vi "Append Dictionary.vi"(8 "error in (no error)":errorcluster, 10 "key-value":T1, 11 "Control Experiment":refnum<class "Control Experiment.lvclass">) -> (0 "error out":errorcluster, 3 "Control Experiment out":refnum<class "Control Experiment.lvclass">)   [LabVIEW 2016, in "Control Experiment.lvclass"]
uses:
  Control Experiment.lvclass
  <userlib>/LevyLab/LV to ITX/Data/Typedefs/Dictionary--cluster.ctl
  <userlib>/LevyLab/LV to ITX/Data/Data.lvclass
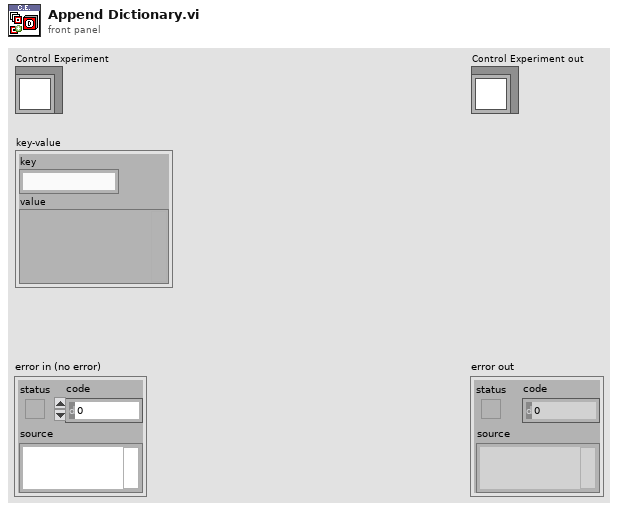
[diagram p1: front panel]
types:
  T1 = typedef "Data.lvclass/Dictionary--cluster.ctl" = cluster{"key":string, "value":variant}
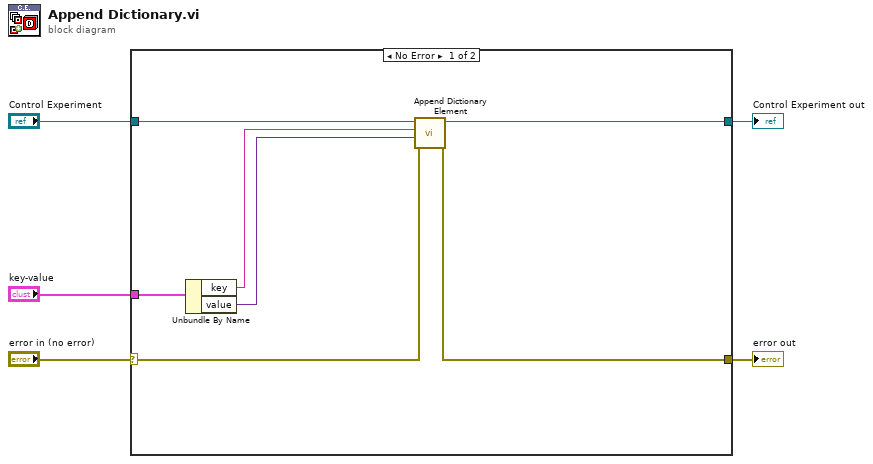
[diagram p0: block diagram]
diagram:
  n1 = case shown="No Error" "error in (no error)" {
    selector: "error in (no error)" -> [w8 w13]
    tunnel: [w7 w13] -> w4
    tunnel: [w6 w14] -> w2
    tunnel: "Control Experiment" -> [w9 w14]
    tunnel: "key-value" -> [w12 _]
    frame No Error {
      n2 = Unbundle By Name(w12) -> ("key"=w10:string, "value"=w11:variant)
      n3 = call "Append Dictionary Element.vi"("error in (no error)"=w8, "value"=w11, "key"=w10, "Control Experiment"=w9) -> ("error out"=w7:errorcluster, "Control Experiment out"=w6:refnum<class "Control Experiment.lvclass">)  [unwired: 6 in]
    }
    frame Error {
    }
  }
  "error out" <- w4
  "Control Experiment out" <- w2
